vi "Write PluginIniFilePath.vi"(8 "error in (no error)":errorcluster, 10 "PluginIniFilePath":path, 11 "BasePlugin in":refnum<class "BasePlugin.lvclass">) -> (0 "error out":errorcluster, 3 "BasePlugin out":refnum<class "BasePlugin.lvclass">)   [LabVIEW 2014, in "BaseClasses.lvlib" / "BasePlugin.lvclass"]
uses:
  BasePlugin.lvclass
  BasePlugin.lvclass/BasePlugin.ctl
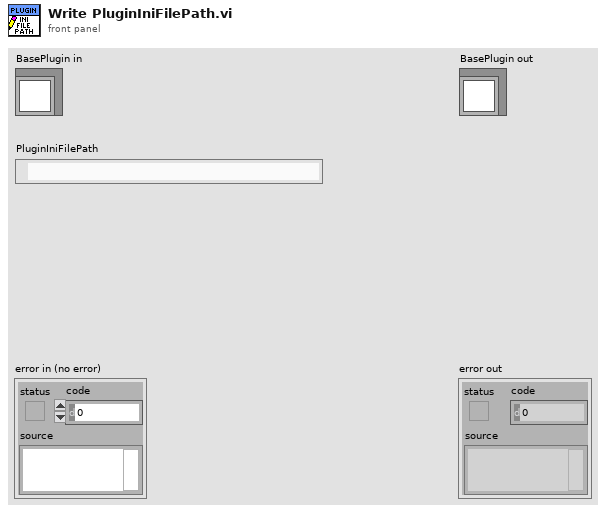
[diagram p1: front panel]
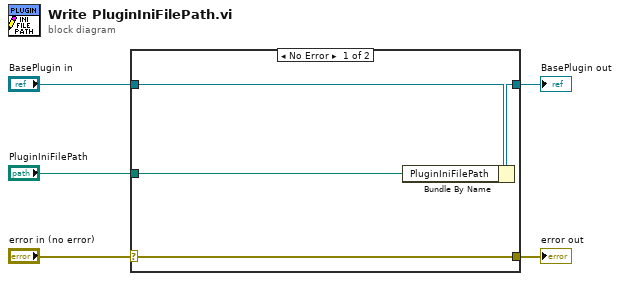
[diagram p0: block diagram]
diagram:
  n1 = case shown="No Error" "error in (no error)" {
    selector: "error in (no error)" -> [w9 w10]
    tunnel: [w9 w10] -> w4
    tunnel: [w7 w11] -> w2
    tunnel: "BasePlugin in" -> [w8 w11]
    tunnel: "PluginIniFilePath" -> [w6 _]
    frame No Error {
      n2 = Bundle By Name(cluster=w8, "PluginIniFilePath"=w6) -> (w7:refnum<class "BasePlugin.lvclass">)
    }
    frame Error {
    }
  }
  "error out" <- w4
  "BasePlugin out" <- w2
